vi "Test using label.vi"() -> ()   [LabVIEW 2020, in "Basic.Mechanics.Tests.lvclass"]
uses:
  Basic.Mechanics.Tests.lvclass
  Source/Approval Tests/Options/Options.lvclass
  Source/Approval Tests/Report Nothing/Report Nothing.lvclass
  C:/Users/SAS/Desktop/ApprovalTests.LabVIEW/Source/Approval Tests/Reporter/Reporter.lvclass
  Source/Approval Tests/Options/Options.lvclass/Options.ctl
  Source/Approval Tests/Naming Data/Naming Data.lvclass/Naming Data.ctl
  9ee2153b-3789-40ef-809e-41e7e893647f.vi
  Source/Approval Tests/Options/Write Reporter.vi
  Source/Approval Tests/Verify Core.vi
  9ee2153b-3789-40ef-809e-41e7e893647f.vi/93c5622b-9fb7-41e0-8c76-3fde37e94e34.vi
  Source/Approval Tests/Update Test Name if Not Defined.vi
  Source/Approval Tests/Options/Read Scrubber.vi
  Source/Approval Tests/Options/Read Namer.vi
  Source/Approval Tests/Options/Read Naming Data.vi
  Source/Approval Tests/Options/Read Reporter.vi
  9ee2153b-3789-40ef-809e-41e7e893647f.vi/93c5622b-9fb7-41e0-8c76-3fde37e94e34.vi/04cb982b-2eda-40d0-8d7e-90f8e0b569b2.vi
  Source/Approval Tests/Naming Data/Read Test VI Name.vi
  Source/Approval Tests/Naming Data/Write Test VI Name.vi
  Source/Approval Tests/Options/Add Label to Namer.vi
  Source/Approval Tests/conv EOL.vi
  <vilib>/Utility/libraryn.llb/Check if File or Folder Exists.vi
  Source/Approval Tests/Reporter/Report.vi
  <vilib>/addons/_JKI Toolkits/Caraya/classes/Assert/Assert False.vi
  <vilib>/addons/_JKI Toolkits/Caraya/classes/Assert/Assert Equal Value_Variant.vi
  Source/Approval Tests/Scrubber/Scrubber.lvclass
  Source/Approval Tests/Namer/Namer.lvclass
  Source/Approval Tests/Naming Data/Naming Data.lvclass
  Source/Approval Tests/Reporter/Reporter.lvclass
  <vilib>/addons/_JKI Toolkits/Caraya/classes/Assert/Assert.lvclass
  <vilib>/addons/_JKI Toolkits/Caraya/classes/Test/Test.lvclass
panel:
  out "Failure Message":string
  out "error out":errorcluster
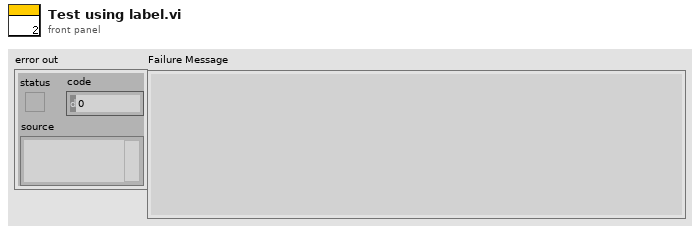
[diagram p1: front panel]
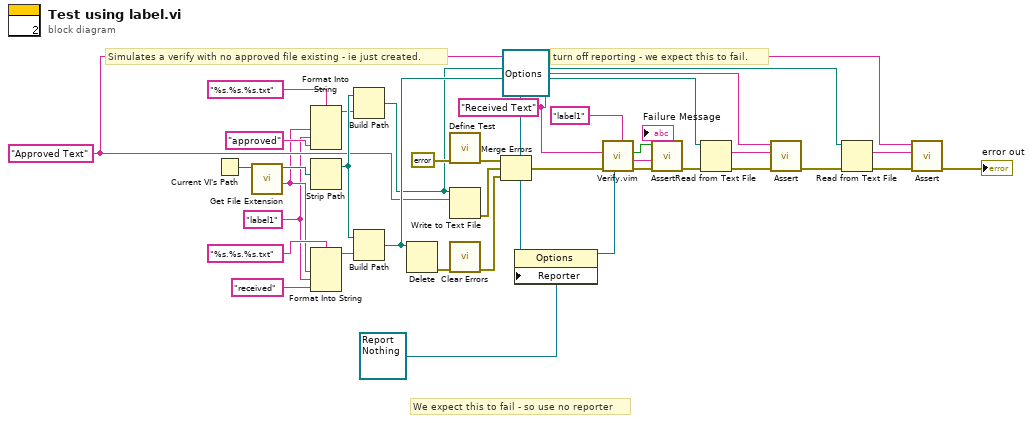
[diagram p0: block diagram]
diagram:
  w10 = "label1" ("input 2")
  w16 = "Approved Text"
  w5 = "Received Text"
  # "We expect this to fail - so use no reporter"
  # "turn off reporting - we expect this to fail."
  # "Simulates a verify with no approved file existing - ie just created."
  n1 = Current VI's Path() -> (path=w33:path)
  n2 = call <vilib>:"Get File Extension.vi"("file"=w33) -> ("filename without extension"=w11:string, "dup file"=w32:path)  [unwired: 6 in, 3 out]
  n3 = Format Into String(format string="%s.%s.%s.txt", w11, w10, "approved" ("string")) -> (resulting string=w12:string)  [unwired: 2 in, 1 out]
  n4 = Strip Path(path=w32) -> (stripped path=w24:path)  [unwired: 1 out]
  n5 = Format Into String(format string="%s.%s.%s.txt", w11, w10, "received" ("string")) -> (resulting string=w8:string)  [unwired: 2 in, 1 out]
  n6 = Build Path(base path=w24, name or relative path=w12) -> (appended path=w17:path)
  n7 = Build Path(base path=w24, name or relative path=w8) -> (appended path=w18:path)
  n8 = Delete(path (use dialog)=w18) -> (error out=w23:errorcluster)  [unwired: 4 in, 2 out]
  n9 = call <vilib>:"Define Test.vi"("error in (no error)"=errorcluster {"status"=FALSE, "code"=0, "source"=""}) -> ("error out"=w19:errorcluster)  [unwired: 9 in, 1 out]
  n10 = Write to Text File(file (use dialog)=w17, text=w16) -> (error out=w22:errorcluster)  [unwired: 2 in, 2 out]
  n11 = call <vilib>:"Clear Errors.vi"("error in (no error)"=w23) -> ("error out"=w21:errorcluster)  [unwired: 5 in, 1 out]
  n12 = Merge Errors(w19, w22, w21) -> (w6:errorcluster)
  n13 = property on="Property Node" class="Options"(reference=refnum<class "Options.lvclass"> refnum ("Options"), "Reporter"=refnum<class "Report Nothing.lvclass"> refnum ("Approval Tests.lvlib:Report Nothing")) -> (reference out=w3:refnum<class "Options.lvclass">)  [unwired: 1 in, 1 out]
  n14 = call "Verify.vim"("Label"="label1", "Options"=w3, "error in"=w6, "Anything"=w5) -> ("error out"=w20:errorcluster, "Failure Message"=→"Failure Message":string, "Passed?"=w34:bool)  [unwired: 5 in]
  n15 = call-poly <vilib>:"Assert.vi"("error in (no error)"=w20, "False?"=w34) -> ("error out"=w31:errorcluster)  [unwired: 8 in, 1 out]
  n16 = Read from Text File(file (use dialog)=w18, error in=w31) -> (text=w28:string, error out=w30:errorcluster)  [unwired: 2 in, 2 out]
  n17 = call-poly <vilib>:"Assert.vi"("error in (no error)"=w30, "Y"=w28, "X"=w5) -> ("error out"=w29:errorcluster)  [unwired: 7 in, 1 out]
  n18 = Read from Text File(file (use dialog)=w17, error in=w29) -> (text=w26:string, error out=w27:errorcluster)  [unwired: 2 in, 2 out]
  n19 = call-poly <vilib>:"Assert.vi"("error in (no error)"=w27, "Y"=w26, "X"=w16) -> ("error out"=→"error out":errorcluster)  [unwired: 7 in, 1 out]
